vi "Baserow Address.vi"(1 "Path":string) -> (0 "URL + Path":string)   [LabVIEW 2018]
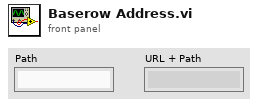
[diagram p1: front panel]
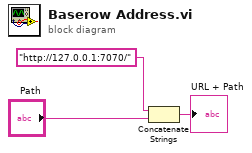
[diagram p0: block diagram]
diagram:
  n1 = Concatenate Strings("http://127.0.0.1:7070/" ("url"), "Path") -> (→"URL + Path":string)
